vi "calculator.vi"() -> ()   [LabVIEW 2021]
panel:
  out "Display":string
  in  "stop":bool
  in  "Calculator Input":T1
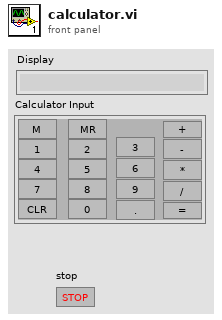
[diagram p1: front panel]
types:
  T1 = cluster{"1":bool, "Add":bool, "Sub":bool, "Multiply":bool, "Divide":bool, "3":bool, "4":bool, "5":bool, "7":bool, "9":bool, "2":bool, "6":bool, "8":bool, "0":bool, "Result":bool, "Clear":bool, "Memory":bool, "Display Memory":bool, "Dicimal":bool}
  T2 = cluster{"A":string, "Operation":string, "Stored":dbl}
  T3 = cluster{"A":string, "Label.Text":string, "Result\n":dbl}
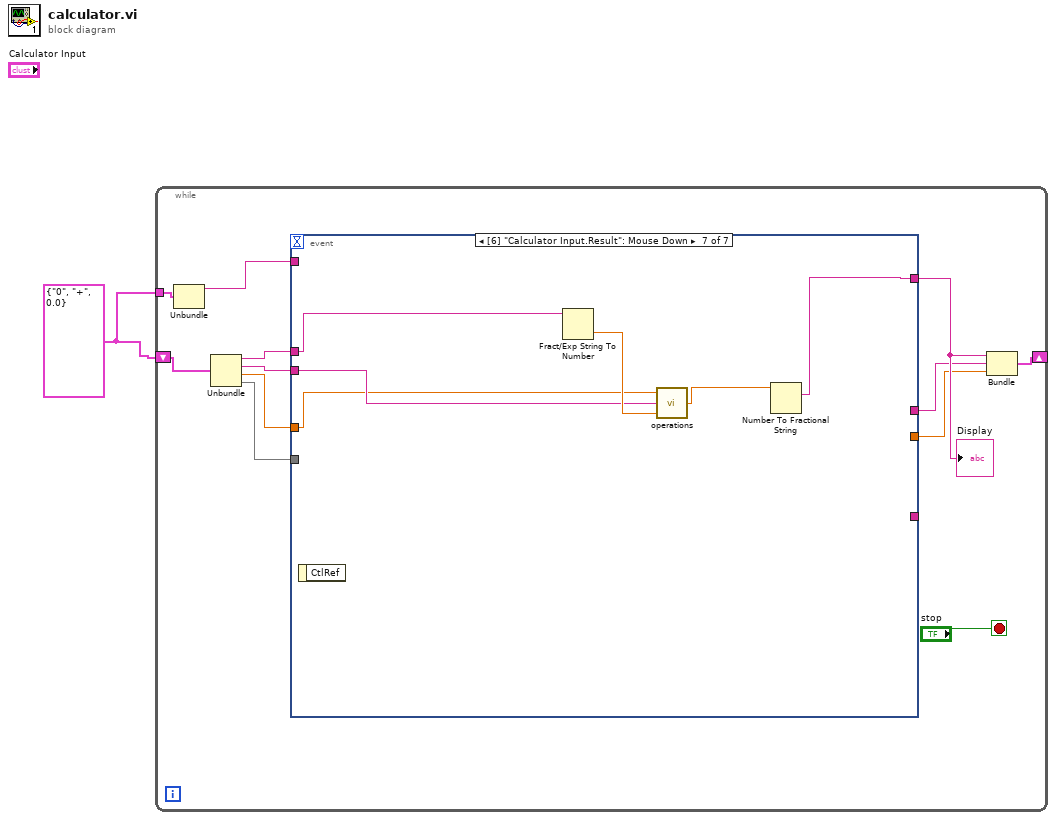
[diagram p0: block diagram]
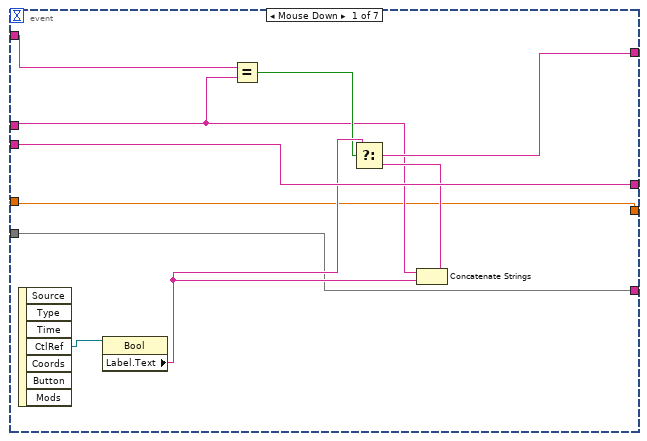
[diagram p2: hidden frame]
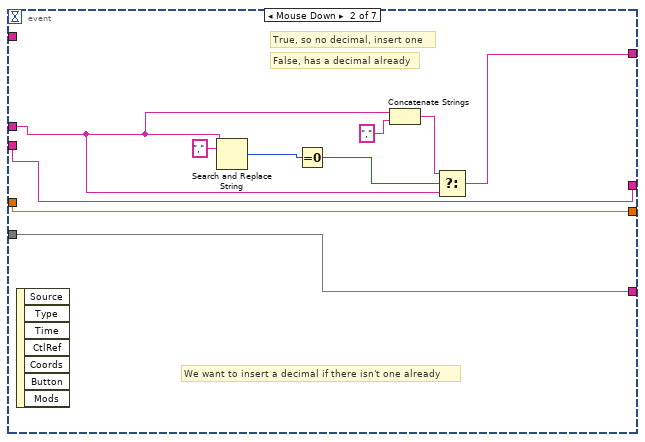
[diagram p3: hidden frame]
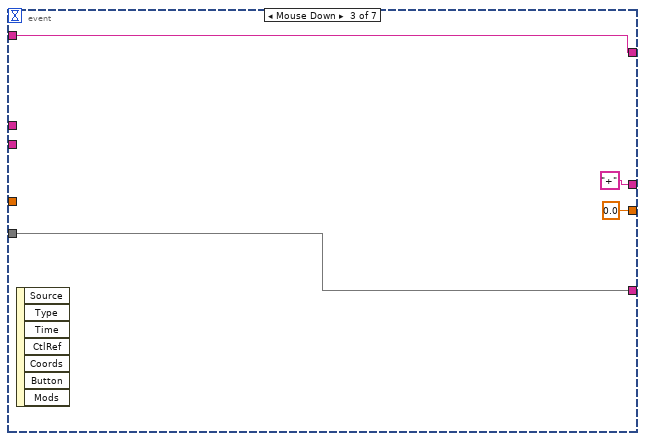
[diagram p4: hidden frame]
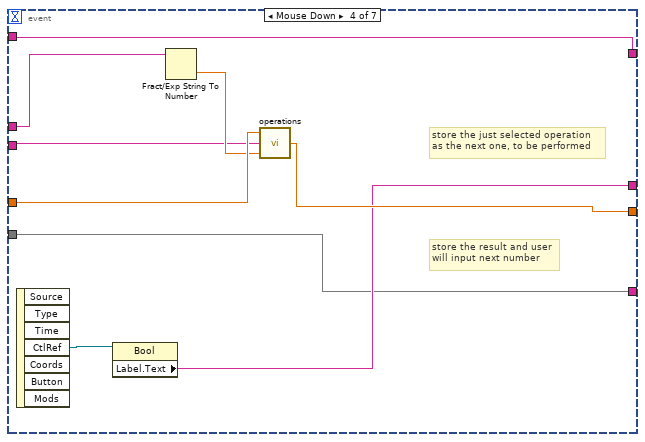
[diagram p5: hidden frame]
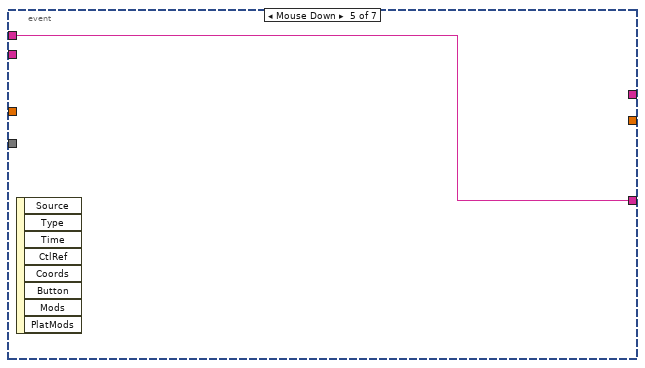
[diagram p6: hidden frame]
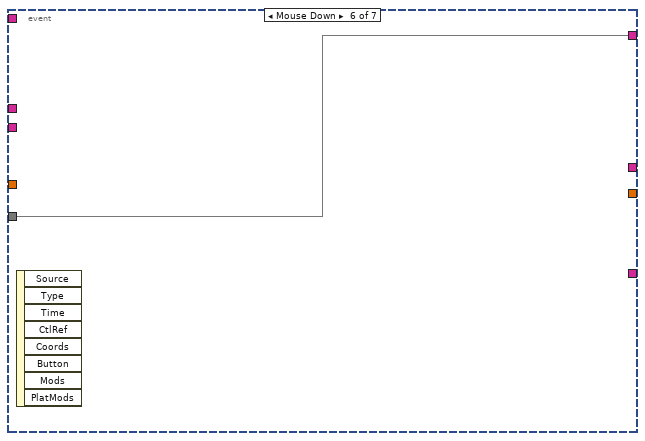
[diagram p7: hidden frame]
diagram:
  w1 = T2 {"A"="0", "Operation"="+", "Stored"=0.0}
  n1 = while {
    shift-right: [w6] -> _
    shift-left: w1 -> [w12]
    tunnel: w1 -> [w9]
    stop <- "stop" stop-if-true
    n2 = Unbundle(w9) -> ("A"=w8:string)  [unwired: 2 out]
    n3 = Unbundle(w12) -> (w11:string, w10:string, w7:dbl, w2)
    n4 = event shown="[6] \"Calculator Input.Result\": Mouse Down" {
      selector: _ -> [_ _ _ _ _ _ _]
      dyn-events: _ -> [_ _ _ _ _ _ _]
      timeout: _ -> [_ _ _ _ _ _ _]
      tunnel: [w19 w30 w35 w41 _ w48 w52] -> w5
      tunnel: w11 -> [w16 w28 _ w43 w47 _ w51]
      tunnel: w10 -> [w22 w25 _ w44 _ _ w50]
      tunnel: [w22 w25 "+" ("Label.Text") w39 _ _ _] -> w4
      tunnel: w8 -> [w17 _ w35 w41 _ _ _]
      tunnel: w7 -> [w15 w26 _ w46 _ _ w49]
      tunnel: [w15 w26 0.0 ("Result") w42 _ _ _] -> w3
      tunnel: w2 -> [w14 w24 w34 w38 _ w48 _]
      tunnel: [w14 w24 w34 w38 w47 _ _] -> _
      event "Calculator Input.0", "Calculator Input.1", "Calculator Input.2", "Calculator Input.3", "Calculator Input.4", "Calculator Input.5", "Calculator Input.6", "Calculator Input.7", "Calculator Input.8", "Calculator Input.9": Mouse Down {
        n5 = event-data() -> ("CtlRef"=w23:refnum<vi>)  [unwired: 1 in, 6 out]
        n6 = property class="Bool"(reference=w23) -> ("Label.Text"=w20:string)  [unwired: 1 in, 2 out]
        n7 = Equal?(x=w17, y=w16) -> (x = y?=w18:bool)
        n8 = Concatenate Strings(w16, w20) -> (w21:string)
        n9 = Select(t=w20, s=w18, f=w21) -> (s? t:f=w19:string)
      }
      event "Calculator Input.Dicimal": Mouse Down {
        # "False, has a decimal already"
        # "True, so no decimal, insert one"
        # "We want to insert a decimal if there isn't one already"
        n10 = event-data() -> ()  [unwired: 1 in, 7 out]
        n11 = Search and Replace String(input string=w28, search string=",") -> (number of replacements=w32:i32)  [unwired: 6 in, 3 out]
        n12 = Equal To 0?(x=w32) -> (x = 0?=w31:bool)
        n13 = Concatenate Strings(w28, "," ("string")) -> (w29:string)
        n14 = Select(t=w29, s=w31, f=w28) -> (s? t:f=w30:string)
      }
      event "Calculator Input.Clear": Mouse Down {
        n15 = event-data() -> ()  [unwired: 1 in, 7 out]
      }
      event "Calculator Input.Add", "Calculator Input.Multiply", "Calculator Input.Sub", "Calculator Input.Divide": Mouse Down {
        # "store the just selected operation\nas the next one, to be performed"
        # "store the result and user\nwill input next number"
        n16 = event-data() -> ("CtlRef"=w40:refnum<vi>)  [unwired: 1 in, 6 out]
        n17 = property class="Bool"(reference=w40) -> ("Label.Text"=w39:string)  [unwired: 1 in, 2 out]
        n18 = Fract/Exp String To Number(string=w43) -> (number=w45:dbl)  [unwired: 3 in, 1 out]
        n19 = call "operations.vi"("B"=w45, "Operation"=w44, "A"=w46) -> ("Result"=w42:dbl)
      }
      event "Calculator Input.Memory": Mouse Down {
        n20 = event-data() -> ()  [unwired: 1 in, 8 out]
      }
      event "Calculator Input.Display Memory": Mouse Down {
        n21 = event-data() -> ()  [unwired: 1 in, 8 out]
      }
      event "Calculator Input.Result": Mouse Down {
        n22 = event-data() -> ()  [unwired: 1 in, 1 out]
        n23 = Fract/Exp String To Number(string=w51) -> (number=w54:dbl)  [unwired: 3 in, 1 out]
        n24 = call "operations.vi"("B"=w54, "Operation"=w50, "A"=w49) -> ("Result"=w53:dbl)
        n25 = Number To Fractional String(number=w53) -> (F-format string=w52:string)  [unwired: 3 in]
      }
    }
    "Display" <- w5
    n26 = Bundle("A"=w5, "Label.Text"=w4, "Result"=w3) -> (w6:T3)  [unwired: 1 in]
  }
